vi "InvertLed.vi"(0 "reference in":refnum<class "LedState.lvclass">, 5 "error in (no error)":errorcluster) -> (14 "reference out":refnum<class "LedState.lvclass">, 19 "error out":errorcluster)   [LabVIEW 2014, in "LedState.lvclass"]
uses:
  LedState.lvclass
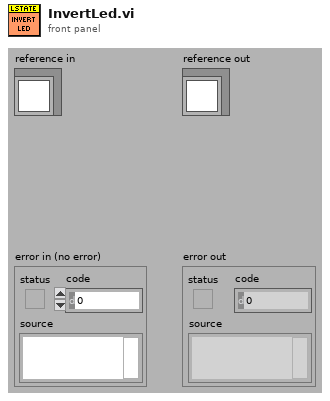
[diagram p1: front panel]
types:
  T1 = typedef "LedState.lvclass/ObjectAttributes.ctl" = cluster{"Led":bool}
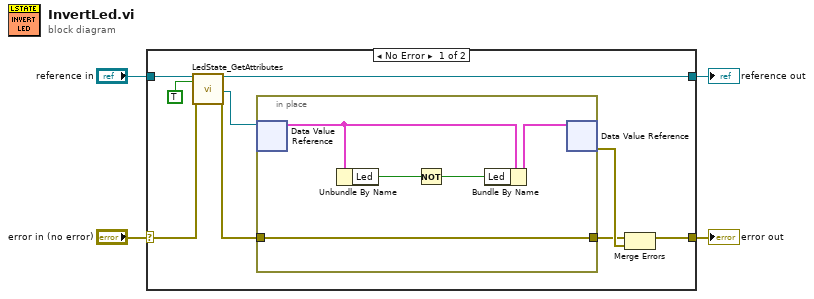
[diagram p0: block diagram]
diagram:
  n1 = case shown="No Error" "error in (no error)" {
    selector: "error in (no error)" -> [w10 w20]
    tunnel: [w12 w20] -> w3
    tunnel: [w8 w19] -> w1
    tunnel: "reference in" -> [w11 w19]
    frame No Error {
      n2 = call "LedState_GetAttributes.vi"("reference in"=w11, "OnlyGetDvrReference(False)"=TRUE, "error in (no error)"=w10) -> ("reference out"=w8:refnum<class "LedState.lvclass">, "DataRef"=w9:refnum<data-value>, "error out"=w6:errorcluster)  [unwired: 13 in, 1 out]
      n3 = in-place {
        in-place-border: w6 -> [w17]
        in-place-border: [w17] -> w5
        n4 = in-place-dvr #1(w9) -> (w16:T1)  [unwired: 1 out]
        n5 = Unbundle By Name(w16) -> ("Led"=w15:bool)
        n6 = Not(x=w15) -> (.not. x?=w14:bool)
        n7 = Bundle By Name(cluster=w16, "Led"=w14) -> (w18:T1)
        n8 = in-place-dvr #1(w18) -> (w13:errorcluster)  [unwired: 1 out]
      }
      n9 = Merge Errors(w5, w13) -> (w12:errorcluster)
    }
    frame Error {
    }
  }
  "error out" <- w3
  "reference out" <- w1
